vi "Ritter Derivative of Totalizer.vi"(8 "error in (no error)":errorcluster, 9 "volume (liters)":dbl, 10 "volume (cuft)":dbl, 11 "timer (hours)":dbl) -> (0 "error out":errorcluster, 2 "Gas Flow Rate (L/hr)-Uncorrected":dbl, 3 "Gas Flow Rate (cuft/hr)-Uncorrected":dbl)   [LabVIEW 2023]
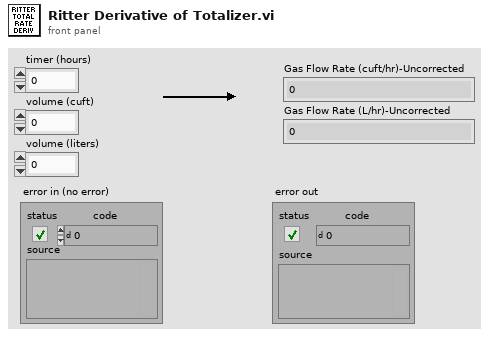
[diagram p1: front panel]
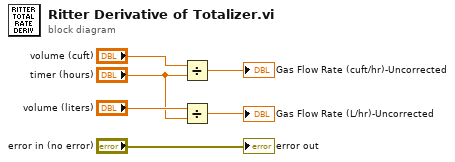
[diagram p0: block diagram]
diagram:
  n1 = Divide(x="volume (cuft)", y="timer (hours)") -> (x/y=→"Gas Flow Rate (cuft/hr)-Uncorrected":dbl)
  n2 = Divide(x="volume (liters)", y="timer (hours)") -> (x/y=→"Gas Flow Rate (L/hr)-Uncorrected":dbl)
  "error out" <- "error in (no error)"
